vi "write_save.vi"(6 "error in":errorcluster, 7 "Difficulty":dbl, 8 "Sequence":dbl[](array[numeric]), 9 "Level":dbl, 10 "Score":dbl, 11 "save file path":path) -> (4 "error out":errorcluster)   [LabVIEW 2024]
uses:
  <vilib>/Utility/config.llb/Write Key (Double).vi
  <vilib>/Utility/config.llb/NI_LVConfig.lvlib
  <vilib>/Utility/config.llb/Write Key (String).vi
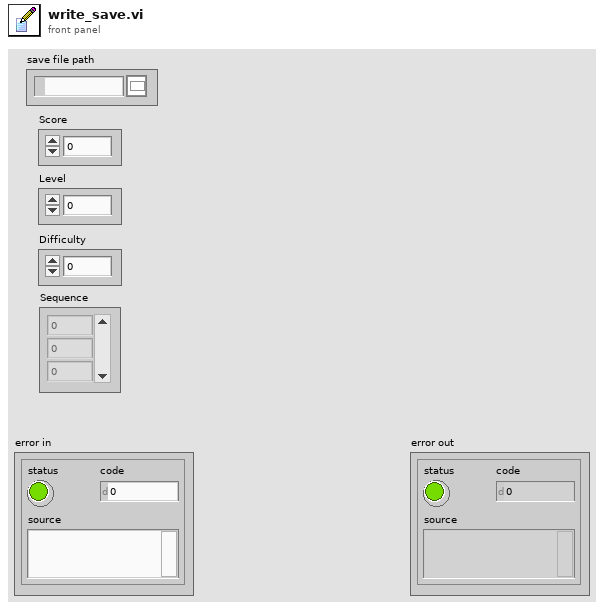
[diagram p1: front panel]
types:
  T1 = typedef "NI_LVConfig.lvlib/Config Data RefNum.ctl" = refnum<k1>
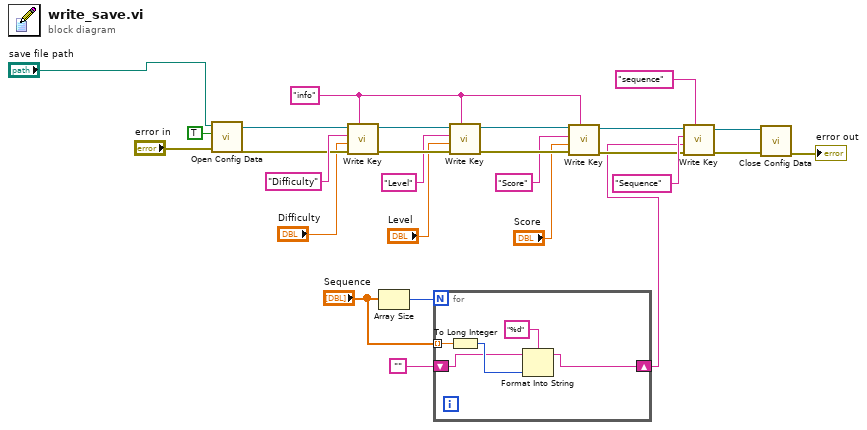
[diagram p0: block diagram]
diagram:
  w16 = "info" ("section")
  n1 = call <vilib>:"Open Config Data.vi"("error in (no error)"="error in", "create file if necessary (T)"=TRUE, "configuration file path"="save file path") -> ("error out"=w23:errorcluster, "refnum"=w24:T1)  [unwired: 6 in, 1 out]
  n2 = call-poly <vilib>:"Write Key.vi"("section"=w16, "error in (no error)"=w23, "value"="Difficulty", "key"="Difficulty", "refnum"=w24) -> ("error out"=w22:errorcluster, "refnum out"=w20:T1)  [unwired: 4 in, 1 out]
  n3 = Array Size(array="Sequence") -> (size(s)=w4:i32)
  n4 = for {
    N: w4 -> [_]
    tunnel: "Sequence" -> [w31] mode=indexing
    shift-right: [w28] -> w1
    shift-left: "" -> [w29]
    n5 = To Long Integer(number=w31) -> (32bit integer=w30:i32)
    n6 = Format Into String(format string="%d", initial string=w29, w30) -> (resulting string=w28:string)  [unwired: 1 in, 1 out]
  }
  n7 = call-poly <vilib>:"Write Key.vi"("section"=w16, "error in (no error)"=w22, "value"="Level", "key"="Level", "refnum"=w20) -> ("error out"=w21:errorcluster, "refnum out"=w19:T1)  [unwired: 4 in, 1 out]
  n8 = call-poly <vilib>:"Write Key.vi"("section"=w16, "error in (no error)"=w21, "value"="Score", "key"="Score", "refnum"=w19) -> ("error out"=w14:errorcluster, "refnum out"=w13:T1)  [unwired: 4 in, 1 out]
  n9 = call-poly <vilib>:"Write Key.vi"("section"="sequence", "error in (no error)"=w14, "value"=w1, "key"="Sequence", "refnum"=w13) -> ("error out"=w10:errorcluster, "refnum out"=w9:T1)  [unwired: 4 in, 1 out]
  n10 = call <vilib>:"Close Config Data.vi"("error in (no error)"=w10, "refnum"=w9) -> ("error out"=→"error out":errorcluster)  [unwired: 8 in, 1 out]
